vi "Close Port.vi"(8 "error in (no error)":errorcluster, 11 "Serial IO in":refnum<class "Serial IO.lvclass">) -> (0 "error out":errorcluster, 3 "Serial IO out":refnum<class "Serial IO.lvclass">)   [LabVIEW 2015, in "Serial IO.lvclass"]
doc: "Close communication to the serial port."
uses:
  Serial IO.lvclass
  Serial IO.lvclass/Serial IO.ctl
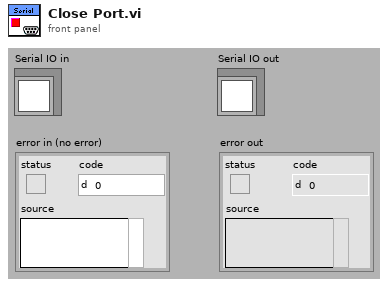
[diagram p1: front panel]
types:
  T1 = typedef "Semaphore RefNum" = refnum<k1>
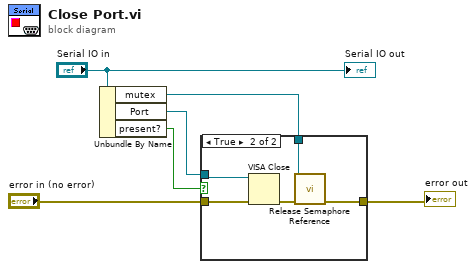
[diagram p0: block diagram]
diagram:
  n1 = Unbundle By Name("Serial IO in") -> ("mutex"=w4:T1, "Port"=w5:refnum<visa-resource-name>, "present?"=w1:bool)
  n2 = case shown="True" w1 {
    tunnel: "error in (no error)" -> [w7 w12]
    tunnel: w5 -> [_ w11]
    tunnel: w4 -> [_ w9]
    tunnel: [w7 w8] -> w3
    frame False {
    }
    frame True {
      n3 = VISA Close(VISA resource name=w11, error in (no error)=w12) -> (error out=w10:errorcluster)
      n4 = call <vilib>:"Release Semaphore Reference.vi"("error in (no error)"=w10, "semaphore"=w9) -> ("error out"=w8:errorcluster)  [unwired: 8 in, 1 out]
    }
  }
  "error out" <- w3
  "Serial IO out" <- "Serial IO in"
